vi "Handle Messages.vi"(8 "error in (no error)":errorcluster, 9 "Message Data":variant, 10 "Message":string, 11 "Customer In":refnum<class "Customer.lvclass">) -> (0 "error out":errorcluster, 3 "Customer Out":refnum<class "Customer.lvclass">)   [LabVIEW 2020, in "Customer.lvclass"]
uses:
  Customer.lvclass
  C:/Users/anton/Documents/GitHub/Triarc-Examples/Coffee Shop/Processes/People/Person/Person.lvclass
  C:/Program Files (x86)/National Instruments/LabVIEW 2020/vi.lib/Asteme/Triarc Framework/Asynchronous Action/Async Action.lvclass
  C:/Program Files (x86)/National Instruments/LabVIEW 2020/vi.lib/Asteme/Triarc Framework/View/View.lvclass
  Support/Beverages/Beverage/Beverage.lvclass
  Customer.lvclass/Customer.ctl
  Support/Beverages/TypeDefs/Drink Type.ctl
  Support/Beverages/TypeDefs/Options.ctl
  Support/Order/Order.lvclass/Order.ctl
  <vilib>/Asteme/Triarc Framework/Process/Process.lvclass/Process.ctl
  <vilib>/Asteme/Triarc Framework/View/View.lvclass/View.ctl
  Process Job/Job Handler.lvclass
  <vilib>/Asteme/Triarc Framework/Process/Protected/Messaging/Enqueue Message.vi
  <vilib>/Asteme/Triarc Framework/View/Public/Get View VI Reference.vi
  <vilib>/Utility/error.llb/Clear Errors.vi
  <vilib>/Asteme/Triarc Framework/Process/Public/Lifecycle/Get Lifecycle State.vi
  <vilib>/AdvancedString/1D String Array to Delimited String.vi
  <vilib>/Asteme/Triarc Framework/Process/Protected/Messaging/Request Message.vi
  <vilib>/Asteme/Triarc Framework/Process/Private/SubVIs/Enqueue Request Message.vi
  <vilib>/Asteme/Triarc Framework/View/View.lvclass
  C:/Program Files (x86)/National Instruments/LabVIEW 2020/vi.lib/Asteme/Triarc Framework/Process/Process.lvclass
  <vilib>/Utility/error.llb/Error Cluster From Error Code.vi
  <vilib>/Asteme/Triarc Framework/Process/Private/SubVIs/Wait for Response Message.vi
  Person/Person.lvclass
  <vilib>/Asteme/Triarc Framework/Process/Process.lvclass
  Support/Order/Order.lvclass
  <vilib>/Asteme/Triarc Framework/Asynchronous Action/Async Action.lvclass
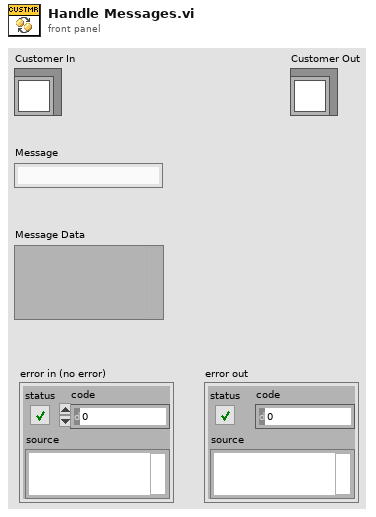
[diagram p1: front panel]
types:
  T1 = typedef "Beverage.lvclass/Drink Type.ctl" = enum16{"Dark Roast", "Decaf", "Espresso", "House Blend"}
  T2 = typedef "Beverage.lvclass/Options.ctl" = enum16{"<None>", "Milk", "Mocha", "Soy", "Whip"}
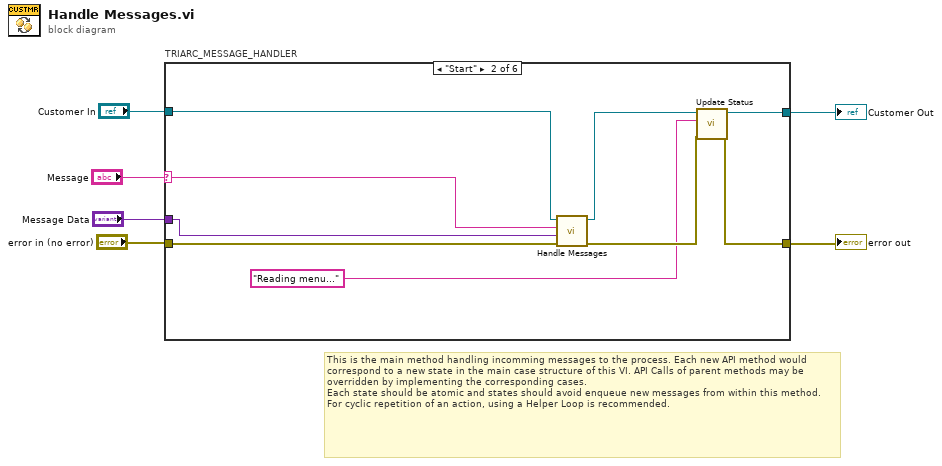
[diagram p0: block diagram]
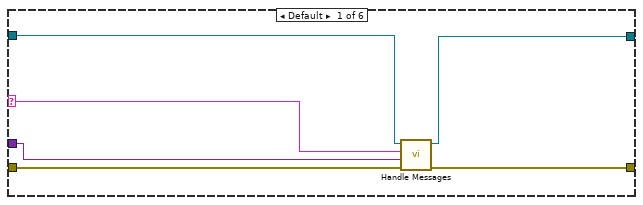
[diagram p2: hidden frame]
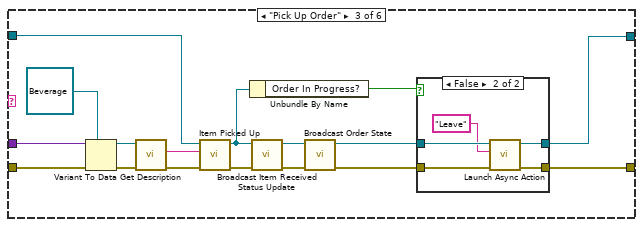
[diagram p3: hidden frame]
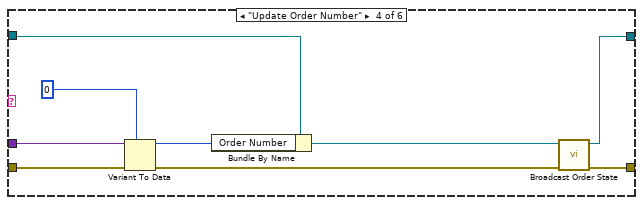
[diagram p5: hidden frame]
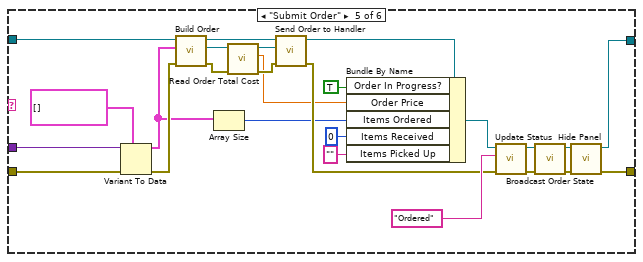
[diagram p6: hidden frame]
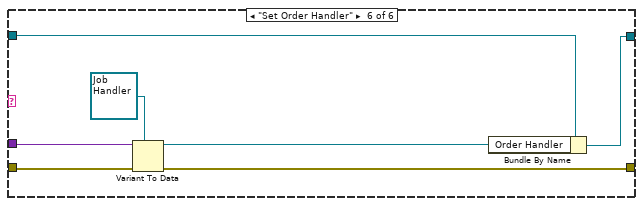
[diagram p7: hidden frame]
diagram:
  # "This is the main method handling incomming messages to the process. Each new API method would correspond to a new state in the main case structure of this VI. API Calls of parent methods may be overridden by implementing the corresponding cases.\nEach state should be atomic and states should avoid enqueue new messages from within this method. For cyclic repetition of an action, using a Helper Loop is recommended."
  n1 = case "TRIARC_MESSAGE_HANDLER" shown="\"Start\"" "Message" {
    selector: "Message" -> [w10 w20 _ _ _ _]
    tunnel: "error in (no error)" -> [w9 w13 w38 w54 w80 w87]
    tunnel: "Customer In" -> [w12 w19 w30 w49 w74 w86]
    tunnel: "Message Data" -> [w11 w21 w37 w52 w79 w82]
    tunnel: [w8 w15 w25 w50 w78 w84] -> w2
    tunnel: [w7 w17 w23 w47 w77 w85] -> w1
    frame Default {
      n2 = call-parent "Handle Messages.vi"("error in (no error)"=w9, "Message Data"=w11, "Message"=w10, "Person In"=w12) -> ("error out"=w8:errorcluster, "Person Out"=w7:refnum<class "Customer.lvclass">)  [unwired: 6 in]
    }
    frame "Start" {
      n3 = call-parent "Handle Messages.vi"("error in (no error)"=w13, "Message Data"=w21, "Message"=w20, "Person In"=w19) -> ("error out"=w16:errorcluster, "Person Out"=w18:refnum<class "Customer.lvclass">)  [unwired: 6 in]
      n4 = call "Update Status.vi"("error in (no error)"=w16, "Status"="Reading menu..." ("Message"), "Person In"=w18) -> ("error out"=w15:errorcluster, "Person Out"=w17:refnum<class "Customer.lvclass">)  [unwired: 7 in]
    }
    frame "Pick Up Order" {
      n5 = Variant To Data(error in=w38, type=refnum<class "Beverage.lvclass"> refnum ("Beverage.lvclass"), Variant=w37) -> (data=w35:refnum<class "Beverage.lvclass">, error out=w34:errorcluster)
      n6 = call "Get Description.vi"("error in"=w34, "Beverage in"=w35) -> ("error out"=w33:errorcluster, "Description"=w29:string)  [unwired: 7 in, 1 out]
      n7 = call "Item Picked Up.vi"("error in (no error)"=w33, "Item Picked Up"=w29, "Customer in"=w30) -> ("error out"=w31:errorcluster, "Customer out"=w26:refnum<class "Customer.lvclass">)  [unwired: 7 in]
      n8 = Unbundle By Name(w26) -> ("Order In Progress?"=w22:bool)
      n9 = call "Broadcast Item Received Status Update.vi"("error in (no error)"=w31, "Customer in"=w26) -> ("error out"=w28:errorcluster, "Customer out"=w27:refnum<class "Customer.lvclass">)  [unwired: 8 in]
      n10 = call "Broadcast Order State.vi"("error in (no error)"=w28, "Customer in"=w27) -> ("error out"=w32:errorcluster, "Customer out"=w24:refnum<class "Customer.lvclass">)  [unwired: 8 in]
      n11 = case shown="False" w22 {
        tunnel: w32 -> [w39 w45]
        tunnel: [w39 w44] -> w25
        tunnel: w24 -> [w40 w43]
        tunnel: [w40 w42] -> w23
        frame True {
        }
        frame False {
          n12 = call <vilib>:"Launch Async Action.vi"("error in (no error)"=w45, "Message"="Leave", "Async Action In"=w43) -> ("error out"=w44:errorcluster, "Async Action Out"=w42:refnum<class "Customer.lvclass">)  [unwired: 7 in]
        }
      }
    }
    frame "Update Order Number" {
      n13 = Variant To Data(error in=w54, type=u32 0 ("Order Number"), Variant=w52) -> (data=w46:u32, error out=w53:errorcluster)
      n14 = Bundle By Name(cluster=w49, "Order Number"=w46) -> (w48:refnum<class "Customer.lvclass">)
      n15 = call "Broadcast Order State.vi"("error in (no error)"=w53, "Customer in"=w48) -> ("error out"=w50:errorcluster, "Customer out"=w47:refnum<class "Customer.lvclass">)  [unwired: 8 in]
    }
    frame "Submit Order" {
      n16 = Variant To Data(error in=w80, type=cluster{"Drink type":T1, "Options":T2[]}[] [] ("Order Content"), Variant=w79) -> (data=w58:cluster{"Drink type":T1, "Options":T2[]}[], error out=w67:errorcluster)
      n17 = call "Build Order.vi"("error in (no error)"=w67, "Order Content"=w58, "Customer In"=w74) -> ("error out"=w63:errorcluster, "Order Out"=w65:refnum<class "Order.lvclass">, "Customer Out"=w68:refnum<class "Customer.lvclass">)  [unwired: 6 in]
      n18 = Array Size(array=w58) -> (size(s)=w57:i32)
      n19 = call "Read Order Total Cost.vi"("error in (no error)"=w63, "Order in"=w65) -> ("error out"=w62:errorcluster, "Order Total Cost"=w61:dbl, "Order out"=w64:refnum<class "Order.lvclass">)  [unwired: 7 in]
      n20 = call "Send Order to Handler.vi"("error in (no error)"=w62, "Order Out"=w64, "Customer In"=w68) -> ("error out"=w73:errorcluster, "Customer Out"=w60:refnum<class "Customer.lvclass">)  [unwired: 7 in]
      n21 = Bundle By Name(cluster=w60, "Order In Progress?"=TRUE ("Order State.Order In Progress?"), "Order Price"=w61, "Items Ordered"=w57, "Items Received"=u32 0 ("Order State.Items Received"), "Items Picked Up"="" ("Order State.Items Picked Up")) -> (w59:refnum<class "Customer.lvclass">)
      n22 = call "Update Status.vi"("error in (no error)"=w73, "Status"="Ordered", "Person In"=w59) -> ("error out"=w72:errorcluster, "Person Out"=w70:refnum<class "Customer.lvclass">)  [unwired: 7 in]
      n23 = call "Broadcast Order State.vi"("error in (no error)"=w72, "Customer in"=w70) -> ("error out"=w71:errorcluster, "Customer out"=w69:refnum<class "Customer.lvclass">)  [unwired: 8 in]
      n24 = call <vilib>:"Hide Panel.vi"("error in (no error)"=w71, "View In"=w69) -> ("error out"=w78:errorcluster, "View Out"=w77:refnum<class "Customer.lvclass">)  [unwired: 8 in]
    }
    frame "Set Order Handler" {
      n25 = Variant To Data(error in=w87, type=refnum<class "Job Handler.lvclass"> refnum ("Job Handler.lvclass"), Variant=w82) -> (data=w83:refnum<class "Job Handler.lvclass">, error out=w84:errorcluster)
      n26 = Bundle By Name(cluster=w86, "Order Handler"=w83) -> (w85:refnum<class "Customer.lvclass">)
    }
  }
  "error out" <- w2
  "Customer Out" <- w1
